vi "List Git Repo Folders_lvcicd.vi"(8 "error in (no error)":errorcluster, 11 "path":path) -> (0 "error out":errorcluster, 3 "Repo Folders":path[](array[path]))   [LabVIEW 2019]
doc: "lvAPT-User-Libraries 2022.4.27.213228\nYAO - lvAPT\nCopyright (c) 2022, lvAPT"
uses:
  <userlib>/_OpenG.lib/file/file.llb/Build Path - File Names Array__ogtk.vi
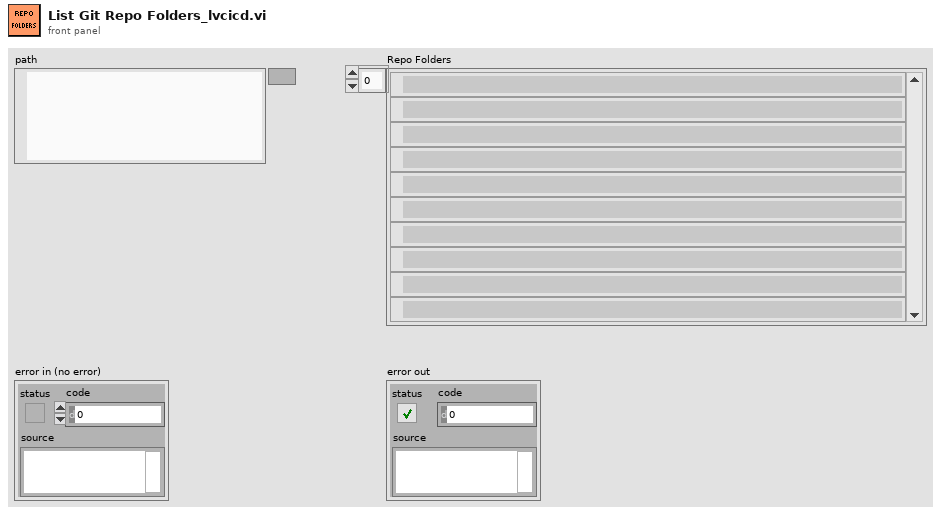
[diagram p1: front panel]
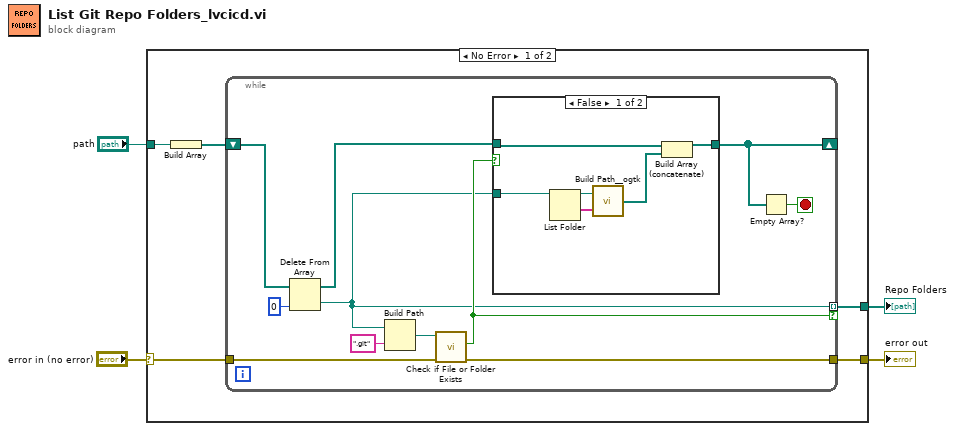
[diagram p0: block diagram]
diagram:
  n1 = case shown="No Error" "error in (no error)" {
    selector: "error in (no error)" -> [w6 w28]
    tunnel: "path" -> [w9 _]
    tunnel: [w7 _] -> w3
    tunnel: [w5 w28] -> w1
    frame No Error {
      n2 = Build Array(w9) -> (w8:path[])
      n3 = while {
        shift-right: [w16] -> _
        shift-left: w8 -> [w13]
        tunnel: [w10] -> w7 mode=indexing if=w18
        tunnel: w6 -> [w15]
        tunnel: [w14] -> w5
        stop <- w17 stop-if-true
        n4 = Delete From Array(array=w13, index=0) -> (deleted portion=w10:path, array with subset deleted=w12:path[])  [unwired: 1 in]
        n5 = Build Path(base path=w10, name or relative path=".git") -> (appended path=w11:path)
        n6 = call <vilib>:"Check if File or Folder Exists.vi"("error in (no error)"=w15, "path"=w11) -> ("error out"=w14:errorcluster, "file or folder exists?"=w18:bool)  [unwired: 7 in, 1 out]
        n7 = case shown="False" w18 {
          tunnel: w12 -> [w23 w27]
          tunnel: w10 -> [w26 _]
          tunnel: [w21 w27] -> w16
          frame False {
            n8 = List Folder(path=w26) -> (path out=w25:path, folder names=w24:string[])  [unwired: 3 in, 2 out]
            n9 = call-poly <userlib>:"Build Path__ogtk.vi"("name or relative path"=w24, "base path"=w25) -> ("appended path"=w22:path[])
            n10 = Build Array (concatenate)(w23, w22) -> (w21:path[])
          }
          frame True {
          }
        }
        n11 = Empty Array?(array=w16) -> (empty?=w17:bool)
      }
    }
    frame Error {
    }
  }
  "Repo Folders" <- w3
  "error out" <- w1
